vi "SJA.vi"(0 "System no.":i32=1 min=1 max=4 step=1, 2 "Axis 1":string, 3 "Axis 2":string, 5 "error in":errorcluster) -> (19 "error out":errorcluster)   [LabVIEW 2026]
doc: "Enables control of the two specified axes with a joystick connected to the controller. Settings will not influence axis settings in Joystick_Operation_Sample_Program.vi which works with a joystick connected to the host computer."
panel:
  # "Enables control of the two specified axes\nwith a joystick connected to the controller."
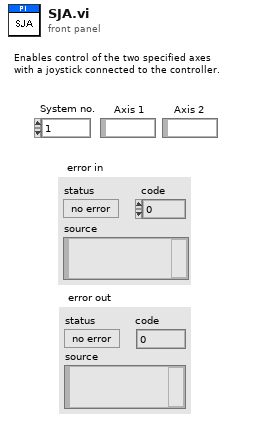
[diagram p1: front panel]
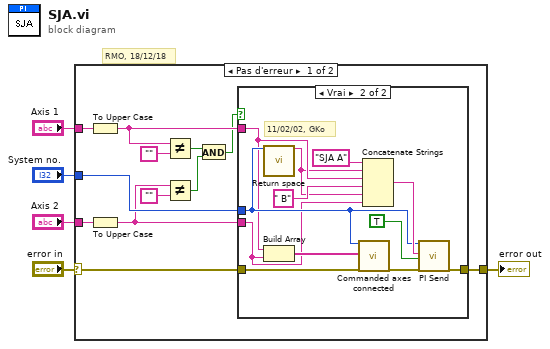
[diagram p0: block diagram]
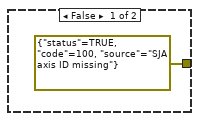
[diagram p2: hidden frame]
diagram:
  # "RMO, 18/12/18"
  n1 = case shown="Pas d'erreur" "error in" {
    selector: "error in" -> [w6 w31]
    tunnel: "Axis 2" -> [w17 _]
    tunnel: "Axis 1" -> [w16 _]
    tunnel: "System no." -> [w15 _]
    tunnel: [w14 w31] -> w2
    frame No Error {
      n2 = To Upper Case(1:w16) -> (0:w13:string)
      n3 = To Upper Case(1:w17) -> (0:w10:string)
      n4 = Not Equal?(x=w13, y="") -> (x != y?=w9:bool)
      n5 = Not Equal?(x=w10, y="") -> (x != y?=w8:bool)
      n6 = And(x=w9, y=w8) -> (x .and. y?=w7:bool)
      n7 = case shown="Vrai" w7 {
        tunnel: w6 -> [_ w27]
        tunnel: w15 -> [_ w23]
        tunnel: [errorcluster {"status"=TRUE, "code"=100, "source"="SJA axis ID missing"} ("error out") w24] -> w14
        tunnel: w13 -> [_ w20]
        tunnel: w10 -> [_ w22]
        frame False {
        }
        frame True {
          # "11/02/02, GKo"
          n8 = call "Return space.vi"("System no."=w23) -> ("String out"=w19:string)  [unwired: 1 in, 17 out]
          n9 = Build Array(w20, w22) -> (w25:string[])
          n10 = call "Commanded axes connected.vi"("System no."=w23, "Commanded axes"=w25, "error in"=w27) -> ("error out"=w26:errorcluster)  [unwired: 1 in, 15 out]
          n11 = Concatenate Strings("SJA A", w19, w20, " B" ("Substring"), w19, w22) -> (w28:string)
          n12 = call "PI Send.vi"("System no."=w23, "String to send"=w28, "Attach termination char.?"=TRUE ("Attach Linefeed?"), "error in"=w26) -> ("error out"=w24:errorcluster)  [unwired: 2 in, 13 out]
        }
      }
    }
    frame Error {
    }
  }
  "error out" <- w2
